vi "credentialCheck.vi"(0 "connection ID in":refnum<k5>, 1 "error in":errorcluster) -> (2 "connection ID out":refnum<k5>, 3 "user":string, 4 "error out":errorcluster)   [LabVIEW 2011]
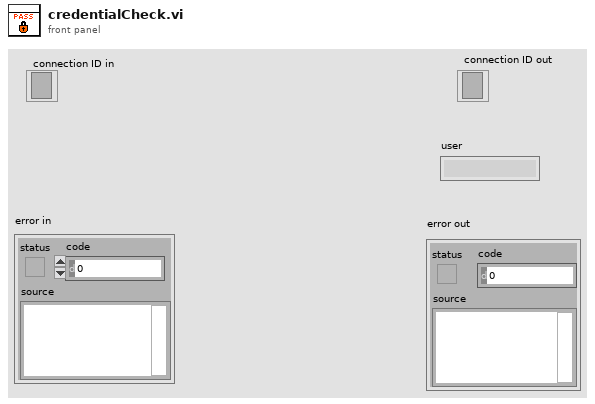
[diagram p1: front panel]
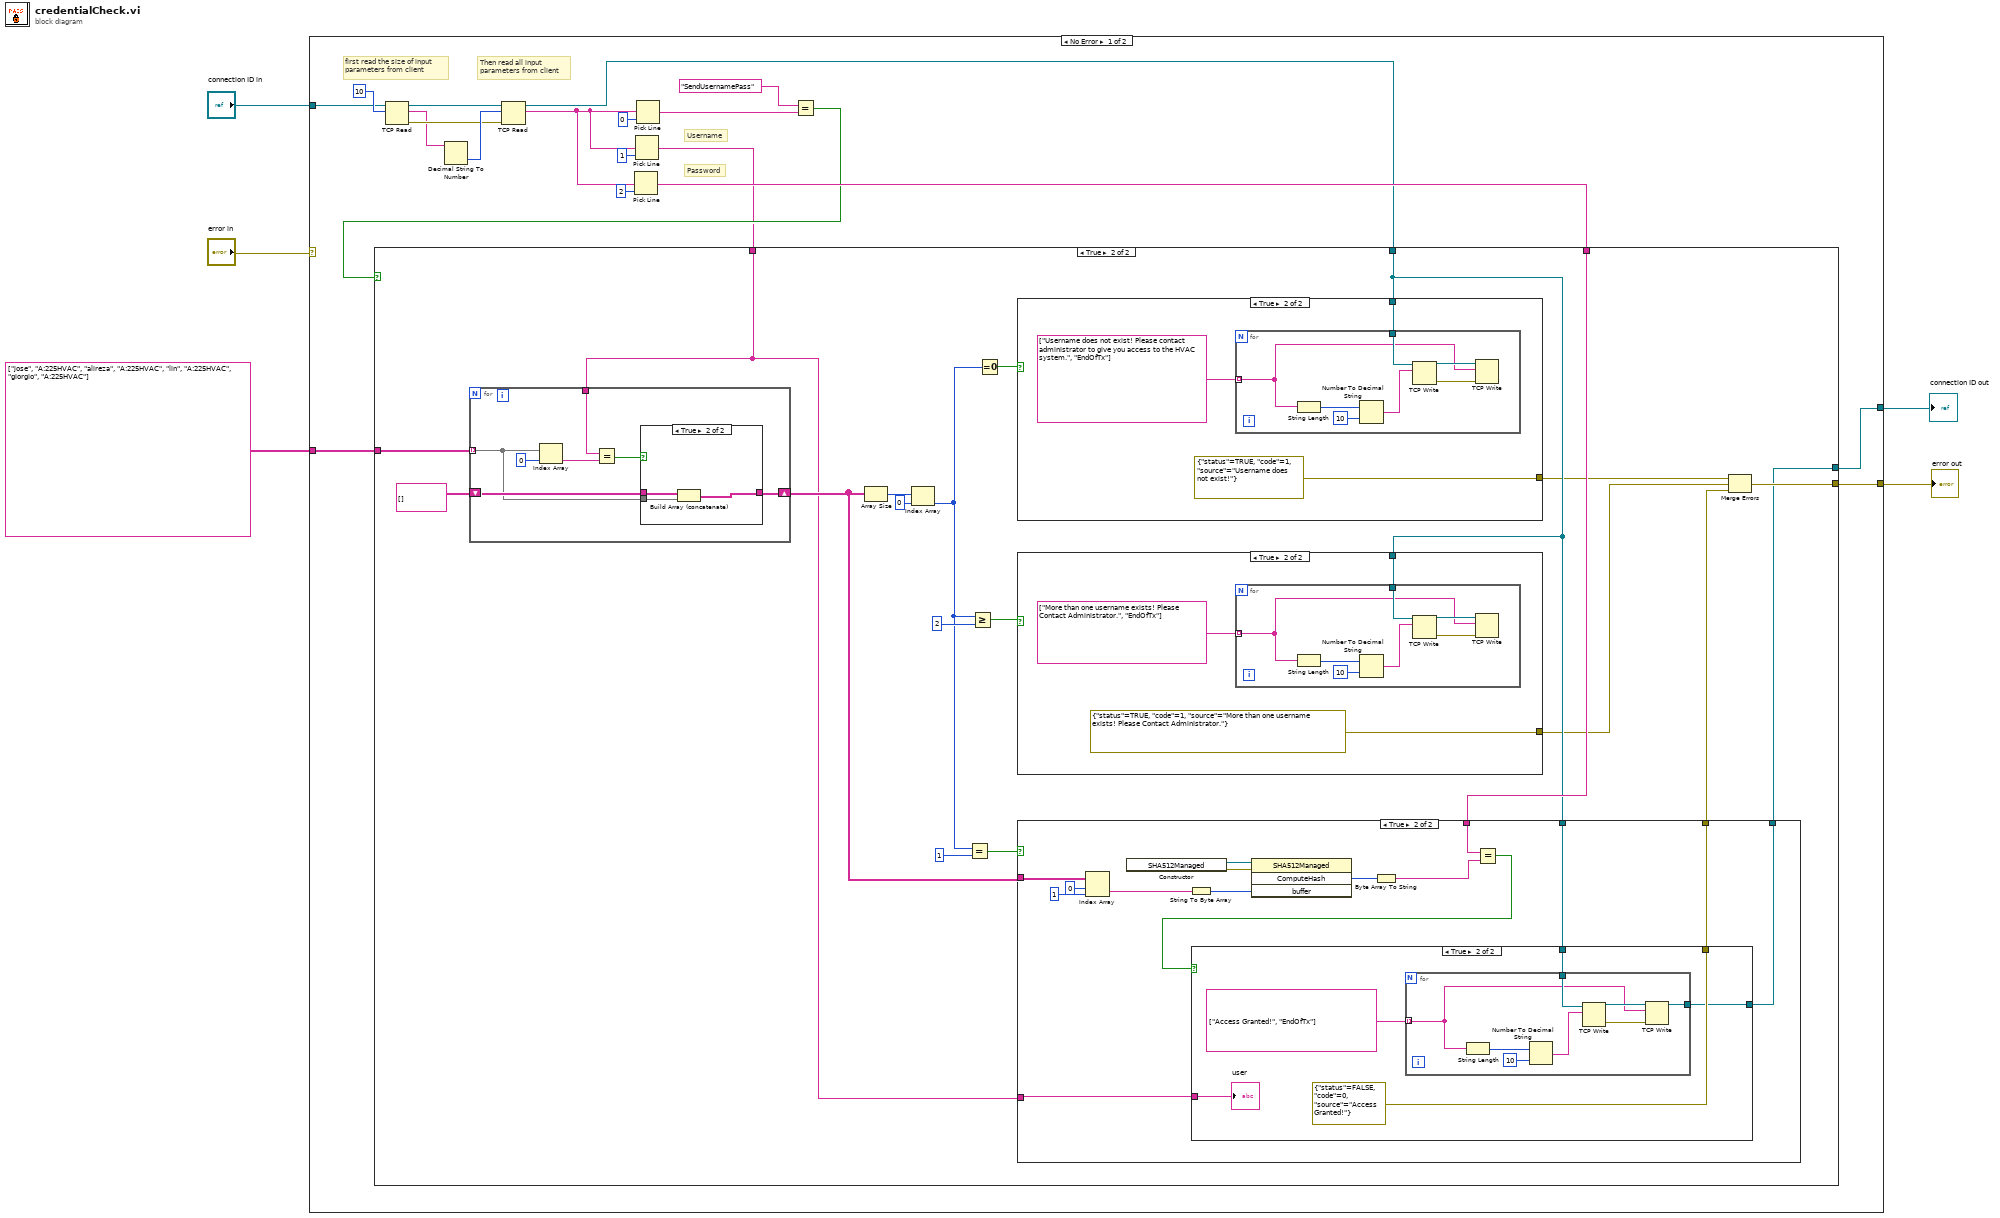
[diagram p0: block diagram]
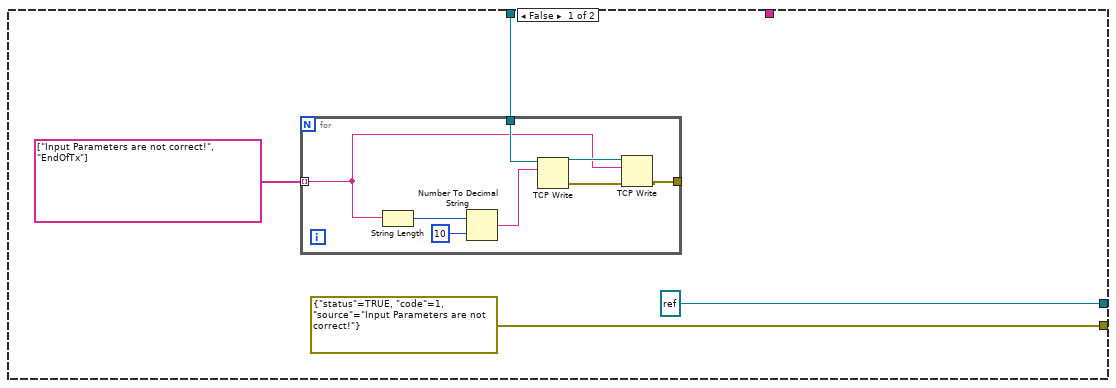
[diagram p2: hidden frame]
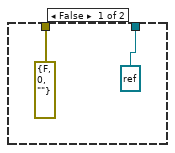
[diagram p3: hidden frame]
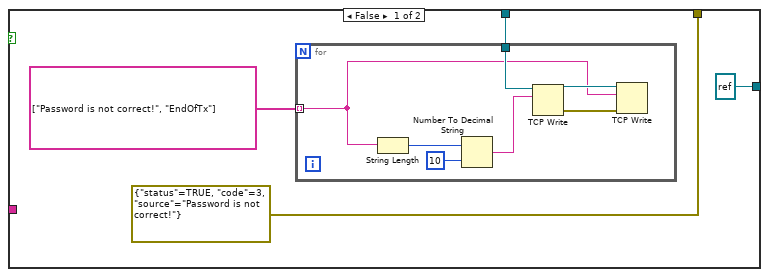
[diagram p4: hidden frame]
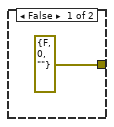
[diagram p5: hidden frame]
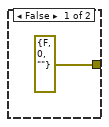
[diagram p6: hidden frame]
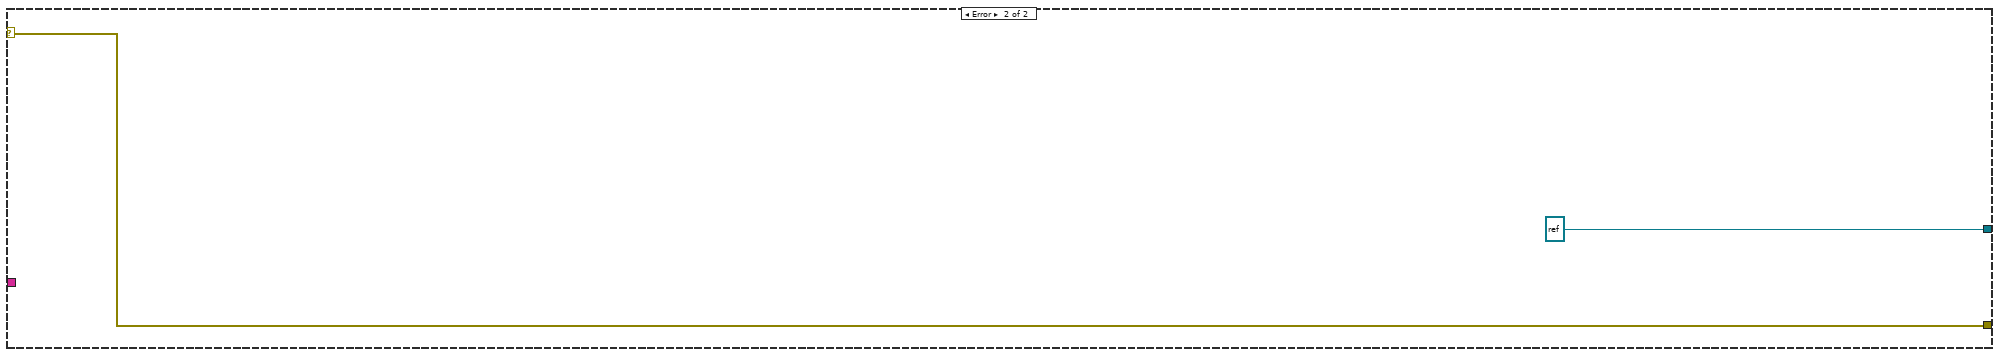
[diagram p8: hidden frame]
diagram:
  n1 = case shown="No Error" "error in" {
    selector: "error in" -> [_ w131]
    tunnel: "connection ID in" -> [w13 _]
    tunnel: [w9 refnum<k5> refnum ("connection ID in")] -> w5
    tunnel: [w10 w131] -> w2
    tunnel: string[][] [["jose", "A:225HVAC"], ["alireza", "A:225HVAC"], ["lin", "A:225HVAC"], ["giorgio", "A:225HVAC"]] -> [w8 _]
    frame No Error {
      # "Then read all input \nparameters from client"
      # "Password"
      # "Username"
      # "first read the size of input \nparameters from client"
      n2 = TCP Read(connection ID=w13, bytes to read=10) -> (connection ID out=w20:refnum<k5>, data out=w19:string, error out=w21:errorcluster)  [unwired: 3 in]
      n3 = Decimal String To Number(string=w19) -> (number=w22:i32)  [unwired: 2 in, 1 out]
      n4 = TCP Read(connection ID=w20, bytes to read=w22, error in (no error)=w21) -> (connection ID out=w6:refnum<k5>, data out=w24:string)  [unwired: 2 in, 1 out]
      n5 = Pick Line(multi-line string=w24, line index=2) -> (output string=w12:string)  [unwired: 1 in]
      n6 = Pick Line(multi-line string=w24, line index=1) -> (output string=w7:string)  [unwired: 1 in]
      n7 = Pick Line(multi-line string=w24, line index=0) -> (output string=w23:string)  [unwired: 1 in]
      n8 = Equal?(x="SendUsernamePass", y=w23) -> (x = y?=w11:bool)
      n9 = case shown="True" w11 {
        tunnel: w12 -> [_ w44]
        tunnel: [errorcluster {"status"=TRUE, "code"=1, "source"="Input Parameters are not correct!"} ("error out") w39] -> w10
        tunnel: [refnum<k5> refnum ("connection ID in") w38] -> w9
        tunnel: w8 -> [_ w54]
        tunnel: w7 -> [_ w37]
        tunnel: w6 -> [w25 w43]
        frame False {
          n10 = for {
            tunnel: w25 -> [w36]
            tunnel: string[] ["Input Parameters are not correct!", "EndOfTx"] -> [w30] mode=indexing
            tunnel: [w29] -> _
            n11 = String Length(string=w30) -> (length=w34:i32)
            n12 = Number To Decimal String(number=w34, width (-)=i16 10) -> (decimal integer string=w33:string)
            n13 = TCP Write(connection ID=w36, data in=w33) -> (connection ID out=w31:refnum<k5>, error out=w32:errorcluster)  [unwired: 2 in, 1 out]
            n14 = TCP Write(connection ID=w31, data in=w30, error in (no error)=w32) -> (error out=w29:errorcluster)  [unwired: 1 in, 2 out]
          }
        }
        frame True {
          n15 = for {
            shift-right: [w119] -> w45
            shift-left: string[][] [] -> [w121]
            tunnel: w54 -> [w120] mode=indexing
            tunnel: w37 -> [w123]
            n16 = Index Array(array=w120, index=0) -> (element=w124:string)
            n17 = Equal?(x=w123, y=w124) -> (x = y?=w122:bool)
            n18 = case shown="True" w122 {
              tunnel: w121 -> [w126 w129]
              tunnel: w120 -> [_ w128]
              tunnel: [w126 w127] -> w119
              frame False {
              }
              frame True {
                n19 = Build Array (concatenate)(w129, w128) -> (w127:string[][])
              }
            }
          }
          n20 = Array Size(array=w45) -> (size(s)=w53:i32[])
          n21 = Index Array(array=w53, index=0) -> (element=w47:i32)
          n22 = Equal?(x=w47, y=1) -> (x = y?=w48:bool)
          n23 = Greater Or Equal?(x=w47, y=2) -> (x >= y?=w49:bool)
          n24 = Equal To 0?(x=w47) -> (x = 0?=w51:bool)
          n25 = case shown="True" w51 {
            tunnel: w43 -> [_ w110]
            tunnel: [errorcluster {"status"=FALSE, "code"=0, "source"=""} ("error out") errorcluster {"status"=TRUE, "code"=1, "source"="Username does not exist!"} ("error out")] -> w42
            frame False {
            }
            frame True {
              n26 = for {
                tunnel: w110 -> [w118]
                tunnel: string[] ["Username does not exist! Please contact administrator to give you access to the HVAC system.", "EndOfTx"] -> [w112] mode=indexing
                n27 = String Length(string=w112) -> (length=w116:i32)
                n28 = Number To Decimal String(number=w116, width (-)=i16 10) -> (decimal integer string=w115:string)
                n29 = TCP Write(connection ID=w118, data in=w115) -> (connection ID out=w113:refnum<k5>, error out=w114:errorcluster)  [unwired: 2 in, 1 out]
                n30 = TCP Write(connection ID=w113, data in=w112, error in (no error)=w114) -> ()  [unwired: 1 in, 3 out]
              }
            }
          }
          n31 = case shown="True" w49 {
            tunnel: w43 -> [_ w99]
            tunnel: [errorcluster {"status"=FALSE, "code"=0, "source"=""} ("error out") errorcluster {"status"=TRUE, "code"=1, "source"="More than one username exists! Please Contact Administrator."} ("error out")] -> w41
            frame False {
            }
            frame True {
              n32 = for {
                tunnel: w99 -> [w107]
                tunnel: string[] ["More than one username exists! Please Contact Administrator.", "EndOfTx"] -> [w101] mode=indexing
                n33 = String Length(string=w101) -> (length=w105:i32)
                n34 = Number To Decimal String(number=w105, width (-)=i16 10) -> (decimal integer string=w104:string)
                n35 = TCP Write(connection ID=w107, data in=w104) -> (connection ID out=w102:refnum<k5>, error out=w103:errorcluster)  [unwired: 2 in, 1 out]
                n36 = TCP Write(connection ID=w102, data in=w101, error in (no error)=w103) -> ()  [unwired: 1 in, 3 out]
              }
            }
          }
          n37 = case shown="True" w48 {
            tunnel: w45 -> [_ w65]
            tunnel: w44 -> [_ w62]
            tunnel: w43 -> [_ w61]
            tunnel: [errorcluster {"status"=FALSE, "code"=0, "source"=""} ("error out") w60] -> w40
            tunnel: [refnum<k5> refnum ("connection ID in") w59] -> w38
            tunnel: w37 -> [_ w58]
            frame False {
            }
            frame True {
              n38 = Index Array(array=w65, index (row)=0 ("index"), index (col)=1 ("disabled index (col)")) -> (element=w63:string)
              n39 = constructor class="SHA512Managed"() -> (reference out=w70:refnum<k24>, error out=w69:errorcluster)  [unwired: 3 in, 1 out]
              n40 = String To Byte Array(string=w63) -> (unsigned byte array=w68:u8[])
              n41 = invoke class="SHA512Managed" method="ComputeHash"(reference=w70, error in=w69, "buffer"=w68) -> ("ComputeHash"=w67:u8[])  [unwired: 1 in, 3 out]
              n42 = Byte Array To String(unsigned byte array=w67) -> (string=w71:string)
              n43 = Equal?(x=w62, y=w71) -> (x = y?=w72:bool)
              n44 = case shown="True" w72 {
                tunnel: w61 -> [w76 w87]
                tunnel: [errorcluster {"status"=TRUE, "code"=3, "source"="Password is not correct!"} ("error out") errorcluster {"status"=FALSE, "code"=0, "source"="Access Granted!"} ("error out")] -> w60
                tunnel: [refnum<k5> refnum ("connection ID in") w85] -> w59
                tunnel: w58 -> [_ w84]
                frame False {
                  n45 = for {
                    tunnel: w76 -> [w83]
                    tunnel: string[] ["Password is not correct!", "EndOfTx"] -> [w77] mode=indexing
                    n46 = String Length(string=w77) -> (length=w81:i32)
                    n47 = Number To Decimal String(number=w81, width (-)=i16 10) -> (decimal integer string=w80:string)
                    n48 = TCP Write(connection ID=w83, data in=w80) -> (connection ID out=w78:refnum<k5>, error out=w79:errorcluster)  [unwired: 2 in, 1 out]
                    n49 = TCP Write(connection ID=w78, data in=w77, error in (no error)=w79) -> ()  [unwired: 1 in, 3 out]
                  }
                }
                frame True {
                  n50 = for {
                    tunnel: w87 -> [w96]
                    tunnel: string[] ["Access Granted!", "EndOfTx"] -> [w90] mode=indexing
                    tunnel: [w89] -> w85
                    n51 = String Length(string=w90) -> (length=w94:i32)
                    n52 = Number To Decimal String(number=w94, width (-)=i16 10) -> (decimal integer string=w93:string)
                    n53 = TCP Write(connection ID=w96, data in=w93) -> (connection ID out=w91:refnum<k5>, error out=w92:errorcluster)  [unwired: 2 in, 1 out]
                    n54 = TCP Write(connection ID=w91, data in=w90, error in (no error)=w92) -> (connection ID out=w89:refnum<k5>)  [unwired: 1 in, 2 out]
                  }
                  "user" <- w84
                }
              }
            }
          }
          n55 = Merge Errors(w42, w41, w40) -> (w39:errorcluster)
        }
      }
    }
    frame Error {
    }
  }
  "connection ID out" <- w5
  "error out" <- w2
